vi "NI9234_SUB-VI_DataStorage.vi"(6 "DataMethod":T1, 8 "error in (no error)":errorcluster, 11 "dataIN":waveform(dbl)[](array[waveform])=[{"t0"=timestamp(0 s since 1904-01-01), "dt"=0.0, "Y"=[1.0, 2.0, 3.0]}, {"t0"=timestamp(0 s since 1904-01-01), "dt"=0.0, "Y"=[4.0, 5.0, 6.0]}, {"t0"=timestamp(0 s since 1904-01-01), "dt"=0.0, "Y"=[7.0, 8.0, 9.0]}, {"t0"=timestamp(0 s since 1904-01-01), "dt"=0.0, "Y"=[11.0, 12.0, 13.0]}]) -> (0 "error out":errorcluster, 2 "size(s)":i32, 3 "DataOUT":dbl[][](array[numeric]))   [LabVIEW 2020]
uses:
  TYPEDEF/NI9234_TD_DataMethod.ctl
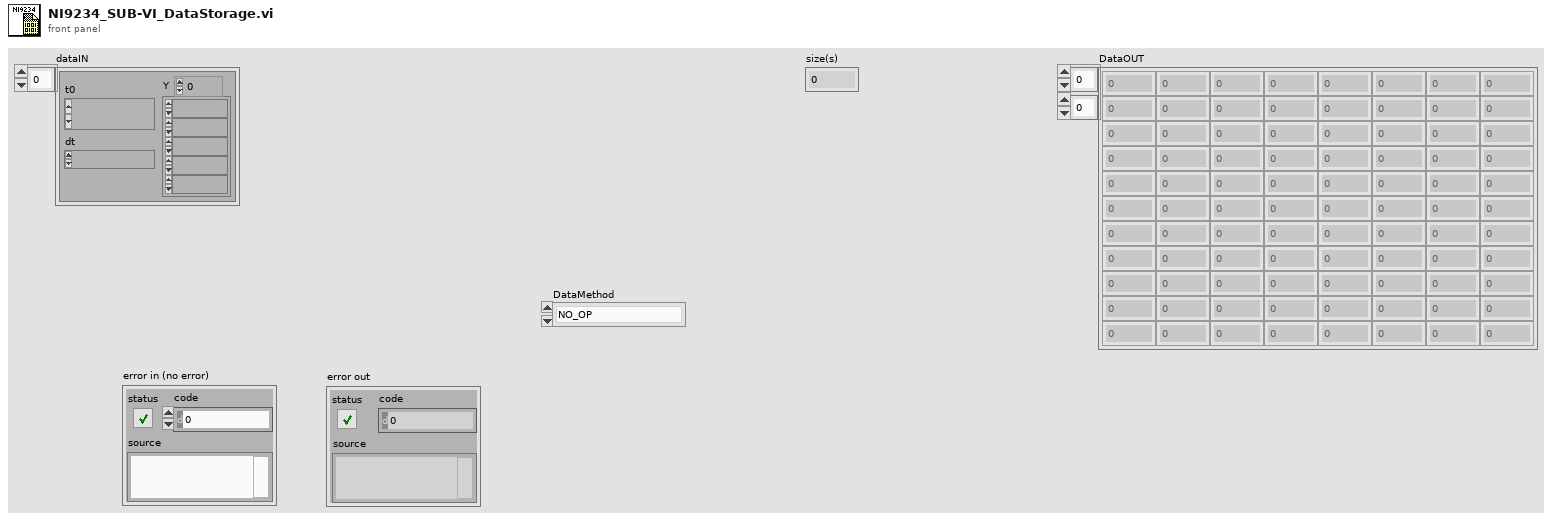
[diagram p1: front panel]
types:
  T1 = typedef "NI9234_TD_DataMethod.ctl" = enum16{"NO_OP", "POPULATE", "USE", "INIT"}
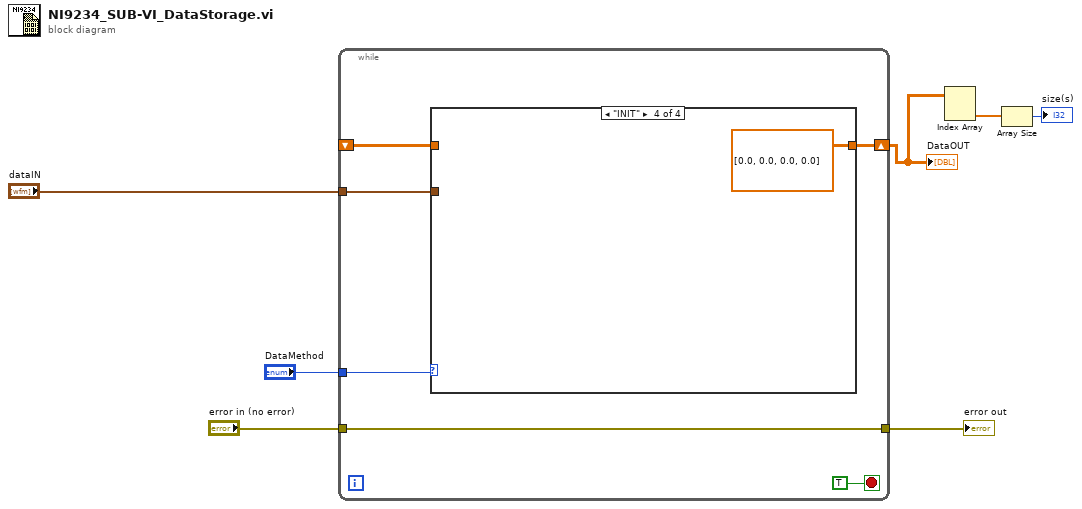
[diagram p0: block diagram]
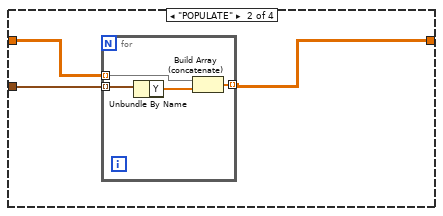
[diagram p3: hidden frame]
diagram:
  n1 = while {
    tunnel: "dataIN" -> [w12]
    tunnel: "DataMethod" -> [w11]
    shift-right: [w10] -> w3
    shift-left: _ -> [w9]
    tunnel: [w8] -> w5
    tunnel: "error in (no error)" -> [w8]
    stop <- TRUE stop-if-true
    n2 = case shown="\"INIT\"" w11 {
      tunnel: w12 -> [_ w17 _ _]
      tunnel: [w14 w15 w22 dbl[][] [[0.0, 0.0, 0.0, 0.0]]] -> w10
      tunnel: w9 -> [w14 w16 w22 _]
      frame "NO_OP", Default {
      }
      frame "POPULATE" {
        n3 = for {
          tunnel: w17 -> [w21] mode=indexing
          tunnel: [w20] -> w15 mode=indexing
          tunnel: w16 -> [w18] mode=indexing
          n4 = Unbundle By Name(w21) -> ("Y"=w19:dbl[])
          n5 = Build Array (concatenate)(w18, w19) -> (w20:dbl[])
        }
      }
      frame "USE" {
      }
      frame "INIT" {
      }
    }
  }
  "DataOUT" <- w3
  "error out" <- w5
  n6 = Index Array(array=w3) -> (element=w2:dbl[])  [unwired: 2 in]
  n7 = Array Size(array=w2) -> (size(s)=→"size(s)":i32)
